vi "Periodic Tasks.vi"() -> ()   [LabVIEW 2011]
doc: "This VI runs in parallel to other tasks. It can contain as many user-defined periodic loops as you need. These can carry out PID or other sorts of timed response."
uses:
  <vilib>/Rock Robotics/SystemInterfaces/Utilities/FPGA_UtilitiesLED State.ctl
  <vilib>/Rock Robotics/SystemInterfaces/Utilities/FPGA_UtilitiesLED Source.ctl
  <vilib>/Rock Robotics/WPI/Relay/WPI_RelayValue.ctl
  Robot Global Data.vi
panel:
  out "Sent?":string="File Wrote"
  out "Voltage":dbl
  in  "Recording Array":dbl[][](array[numeric])
  in  "Turn on Record 2":bool
  out "Auton Recording 2":bool
  in  "Home Speed 2":dbl=1.0
  out "Ramp ACT Pot 2":dbl
  out "Auton Recording":bool
  in  "Turn on Record":bool
  in  "Auton Array":dbl[][](array[numeric])
  out "Right Rate":dbl
  out "Right Direction":bool
  out "Right Distance":dbl
  out "Shooter Encoder Distance":dbl
  out "Shooter Direction":bool
  out "Shooter Encoder Rate":dbl
  out "Left Rate":dbl
  out "Gyro Rate":dbl
  out "Gyro Angle":dbl
  out "Left Direction":bool
  out "Left Distance":dbl
  # "Auton Recording"
  # "Sensor Feedback"
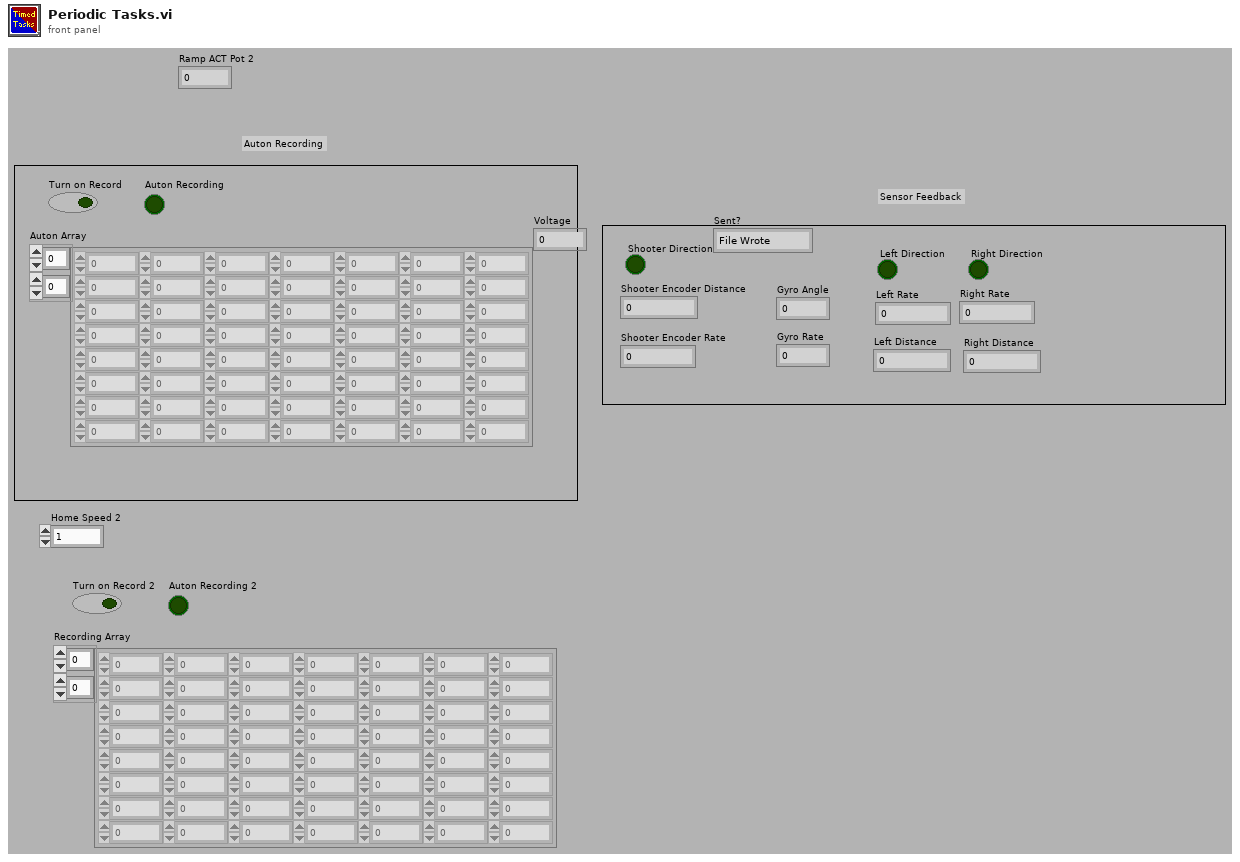
[diagram p1: front panel]
types:
  T1 = typedef "WPI_RelayValue.ctl" = enum16{"Off", "On", "Forward", "Reverse"}
  T2 = cluster{"Driver Station Digital Input (1-8)[0]":bool, "Driver Station Digital Input (1-8)[1]":bool, "Driver Station Digital Input (1-8)[2]":bool, "Driver Station Digital Input (1-8)[3]":bool, "Driver Station Digital Input (1-8)[4]":bool, "Driver Station Digital Input (1-8)[5]":bool, "Driver Station Digital Input (1-8)[6]":bool, "Driver Station Digital Input (1-8)[7]":bool, "Driver Station Digital Input (1-8)[8]":bool}
  T3 = typedef "WPI_AnalogChannelDevRef.ctl" = cluster{"DevStatus":errorcluster, "Analog Module":T4, "Analog Channel":T5}
  T4 = typedef "FPGA_TypedefAnalogModule.ctl" = enum16{"Analog Module 1", "Analog Module 2"}
  T5 = typedef "FPGA_AIChannel.ctl" = enum8{"AI 1", "AI 2", "AI 3", "AI 4", "AI 5", "AI 6", "AI 7", "AI 8", "Invalid"}
  T6 = typedef "WPI_EncoderDevRef.ctl" = cluster{"DevStatus":errorcluster, "EncoderIndex":T7, "CounterIndex":T8, "DistancePerCount":dbl, "Decoding Type":T9}
  T7 = typedef "FPGA_EncoderIdx.ctl" = enum8{"Enc 0", "Enc 1", "Enc 2", "Enc 3", "Invalid"}
  T8 = typedef "FPGA_CounterCtrSystemIndex.ctl" = enum8{"Ctr 0", "Ctr 1", "Ctr 2", "Ctr 3", "Ctr 4", "Ctr 5", "Ctr 6", "Ctr 7", "Invalid"}
  T9 = typedef "WPI_EncoderType.ctl" = enum16{"1x", "2x", "4x"}
  T10 = typedef "WPI_GyroDevRef.ctl" = cluster{"DevStatus":errorcluster, "Analog Module":T4, "Analog Channel":T5, "Offset":dbl, "Gain (VoltsPerDegree/Second)":dbl}
  T11 = typedef "WPI_RelayDevRef.ctl" = cluster{"DevStatus":errorcluster, "Relay Channel":T12, "Digital Module":T13, "Relay Direction":T14}
  T12 = typedef "FPGA_DIORelayChannel.ctl" = enum8{"Relay 1", "Relay 2", "Relay 3", "Relay 4", "Relay 5", "Relay 6", "Relay 7", "Relay 8", "Invalid"}
  T13 = typedef "FPGA_TypedefDigitalModule.ctl" = enum16{"Digital Module 1", "Digital Module 2"}
  T14 = typedef "WPI_RelayDirection.ctl" = enum16{"Both directions", "Forward only", "Reverse only"}
  T15 = typedef "FPGA_UtilitiesLED State.ctl" = enum16{"Off", "On", "Toggle"}
  T16 = typedef "FPGA_UtilitiesLED Source.ctl" = enum16{"User LED", "FPGA LED"}
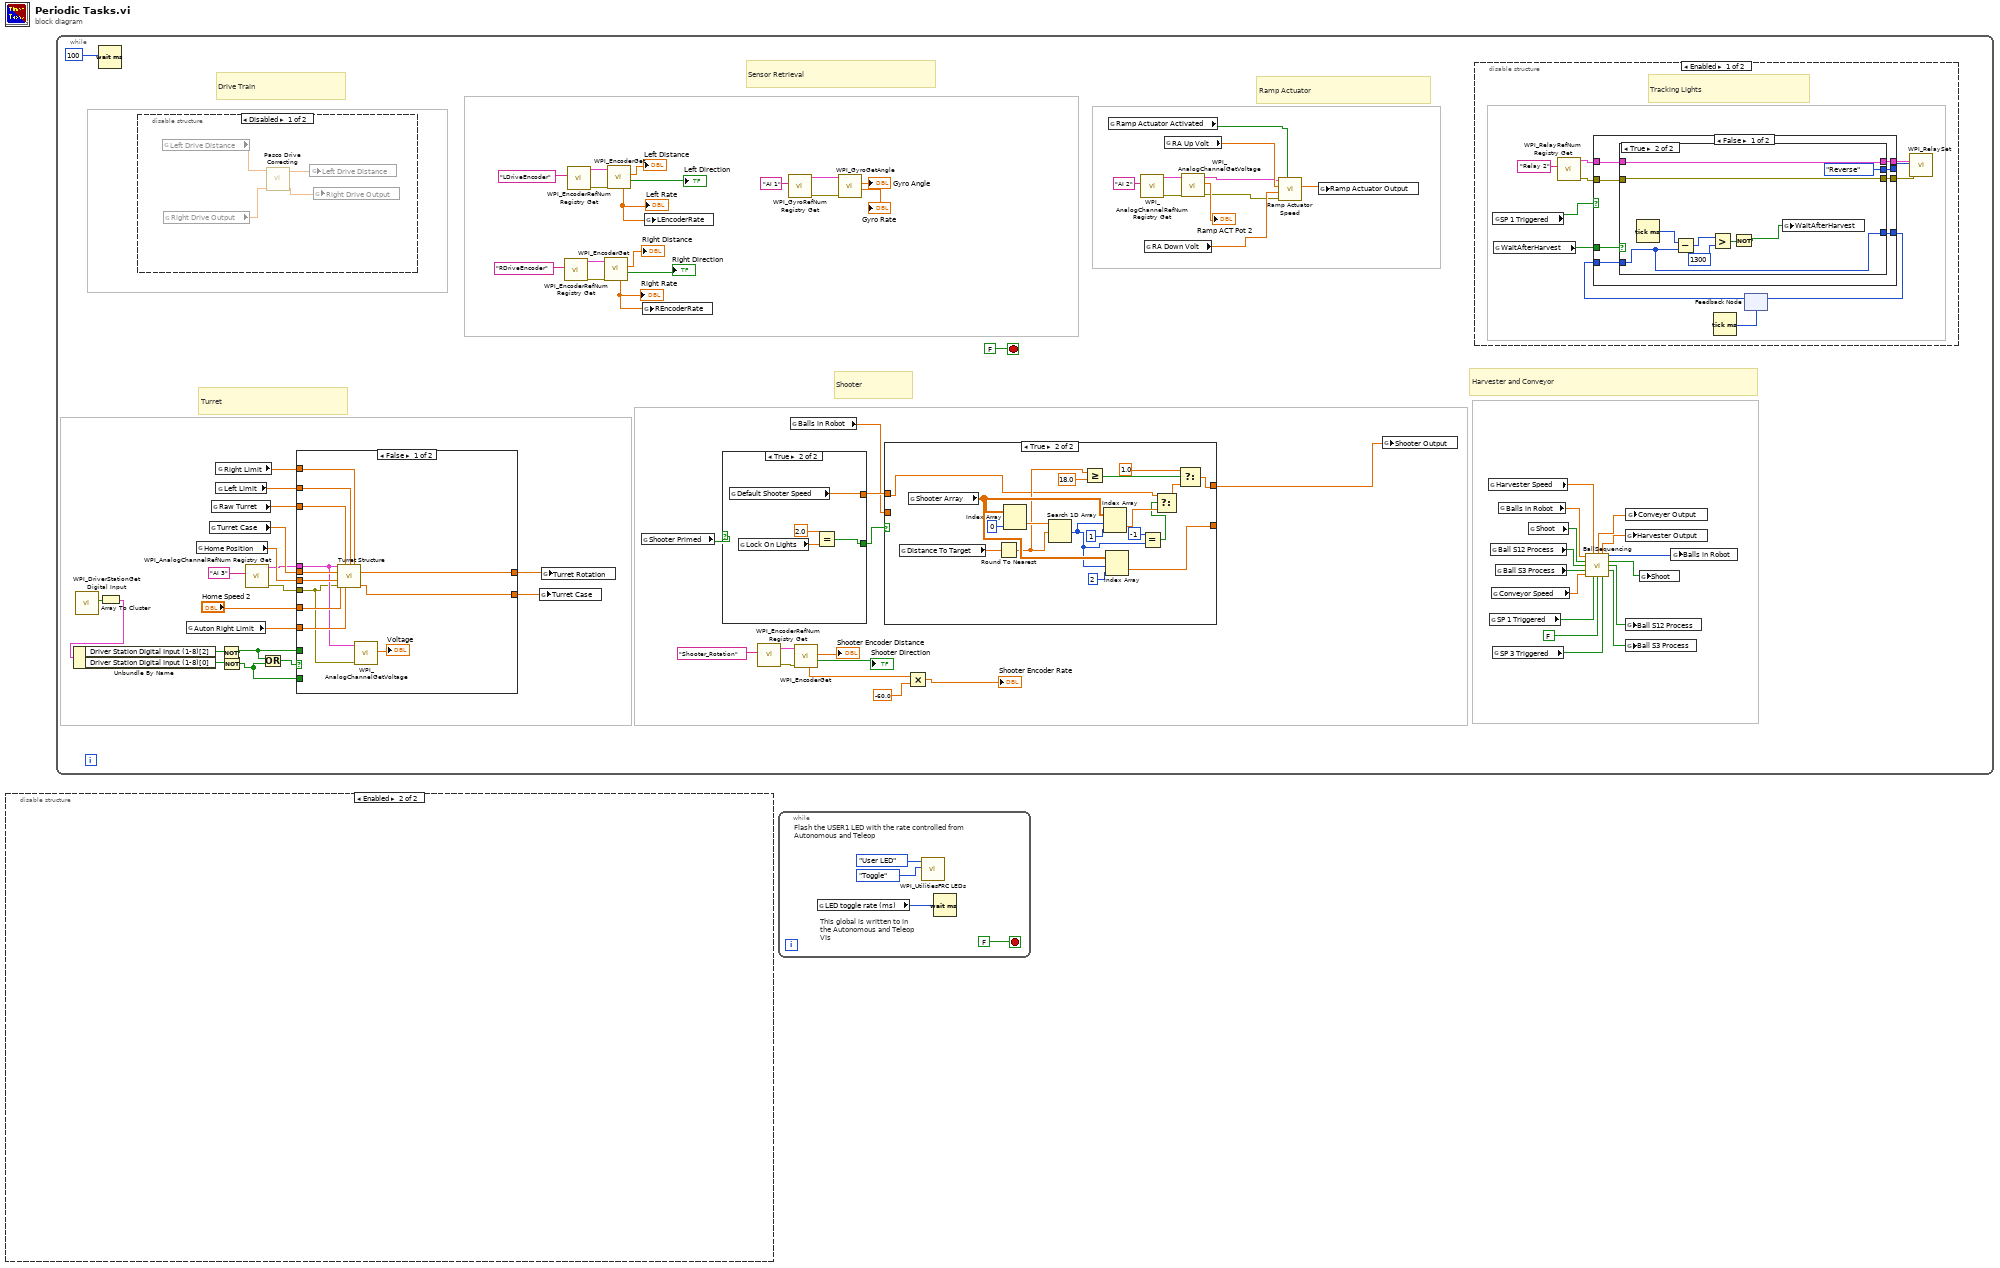
[diagram p0: block diagram]
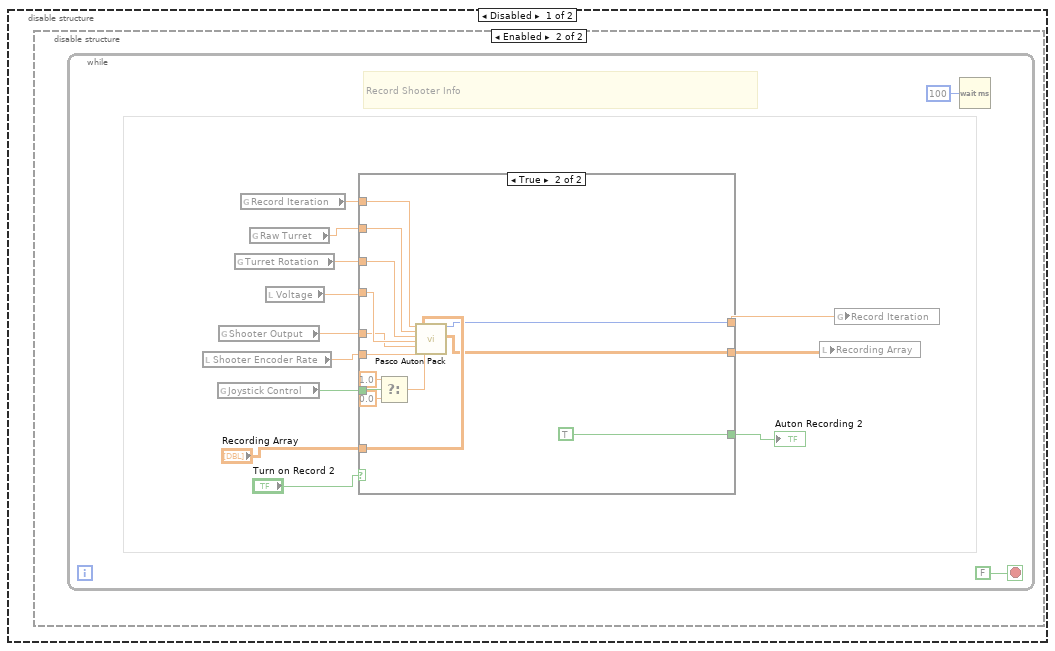
[diagram p2: hidden frame]
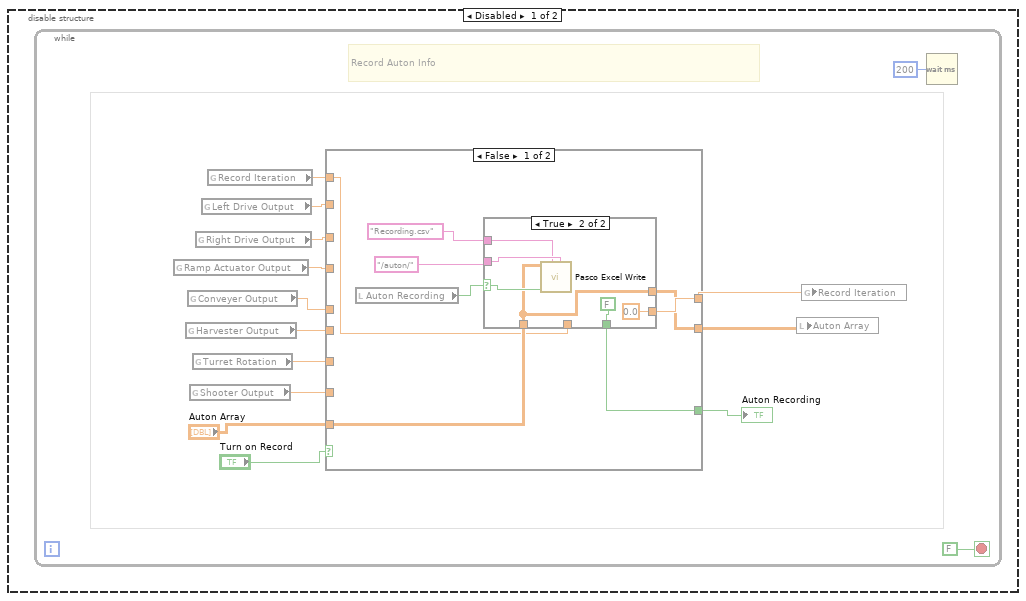
[diagram p3: hidden frame]
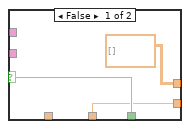
[diagram p4: hidden frame]
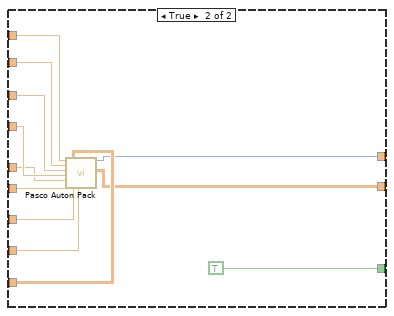
[diagram p5: hidden frame]
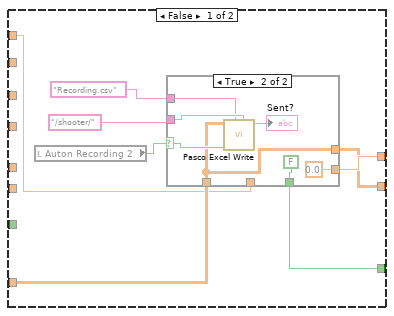
[diagram p6: hidden frame]
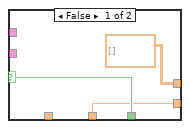
[diagram p7: hidden frame]
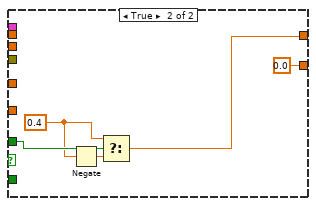
[diagram p8: hidden frame]
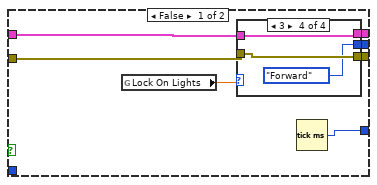
[diagram p9: hidden frame]
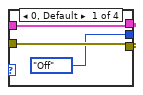
[diagram p10: hidden frame]
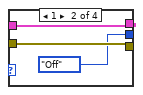
[diagram p11: hidden frame]
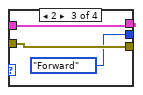
[diagram p12: hidden frame]
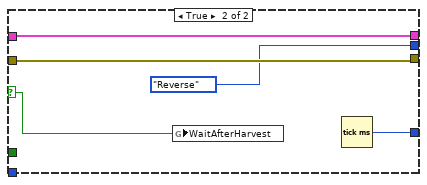
[diagram p13: hidden frame]
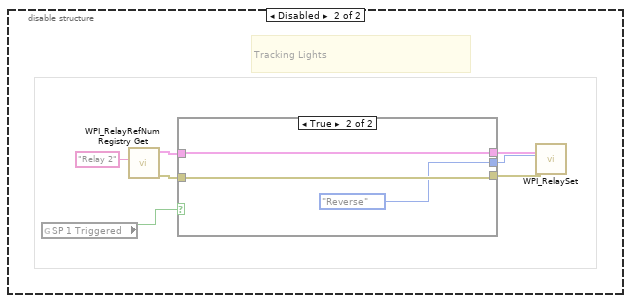
[diagram p14: hidden frame]
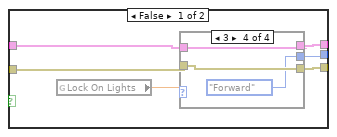
[diagram p15: hidden frame]
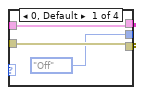
[diagram p16: hidden frame]
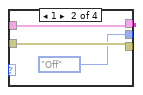
[diagram p17: hidden frame]
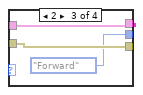
[diagram p18: hidden frame]
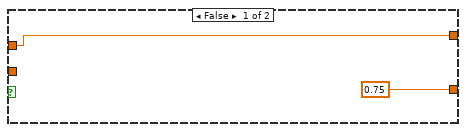
[diagram p19: hidden frame]
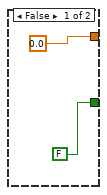
[diagram p20: hidden frame]
diagram:
  n1 = disable-structure shown="Enabled" {
    frame Disabled {
      n2 = disable-structure shown="Enabled" {
        frame Disabled {
          n3 = while {
            stop <- FALSE stop-if-true
            # "Record Auton Info"
            n4 = global read "Robot Global Data.vi" "Ramp Actuator Output"() -> (w5:dbl)
            n5 = global read "Robot Global Data.vi" "Harvester Output"() -> (w7:dbl)
            n6 = global read "Robot Global Data.vi" "Conveyer Output"() -> (w6:dbl)
            n7 = global read "Robot Global Data.vi" "Shooter Output"() -> (w9:dbl)
            n8 = global read "Robot Global Data.vi" "Turret Rotation"() -> (w8:dbl)
            n9 = global read "Robot Global Data.vi" "Right Drive Output"() -> (w4:dbl)
            n10 = global read "Robot Global Data.vi" "Left Drive Output"() -> (w3:dbl)
            n11 = global read "Robot Global Data.vi" "Record Iteration"() -> (w2:dbl)
            n12 = case shown="False" "Turn on Record" {
              tunnel: w2 -> [w19 w44]
              tunnel: w3 -> [_ w43]
              tunnel: w4 -> [_ w42]
              tunnel: w5 -> [_ w41]
              tunnel: w6 -> [_ w40]
              tunnel: w7 -> [_ w39]
              tunnel: w8 -> [_ w38]
              tunnel: w9 -> [_ w37]
              tunnel: "Auton Array" -> [w20 w36]
              tunnel: [w16 w35] -> w12
              tunnel: [w17 w34] -> w13
              tunnel: [w18 TRUE] -> w14
              frame False {
                n13 = local read "Auton Recording"() -> (w21:bool)
                n14 = case shown="True" w21 {
                  selector: w21 -> [w26 w31]
                  tunnel: [w26 FALSE] -> w18
                  tunnel: "/auton/" ("File Name") -> [_ w30]
                  tunnel: "Recording.csv" ("Folder Location") -> [_ w29]
                  tunnel: [w25 0.0 ("Record Iteration")] -> w17
                  tunnel: w19 -> [w25 _]
                  tunnel: w20 -> [_ w27]
                  tunnel: [dbl[][] [] ("Auton Array") w27] -> w16
                  frame False {
                  }
                  frame True {
                    n15 = call "Pasco Excel Write.vi"("Folder Location"=w30, "File Name"=w29, "WriteToExcel"=w31, "2D data"=w27) -> ()  [unwired: 7 in, 1 out]
                  }
                }
              }
              frame True {
                n16 = call "Pasco Auton Pack.vi"("Iterations"=w44, "Left Drive"=w43, "Right Drive"=w42, "RAMP ACT"=w41, "Conveyor"=w40, "Harvestor"=w39, "Auton Array"=w36, "Turret"=w38, "Shooter"=w37) -> ("Iteration Output"=w34:i32, "output array"=w35:dbl[][])  [unwired: 9 in]
              }
            }
            "Auton Recording" <- w14
            n17 = local write "Auton Array"(w12) -> ()
            n18 = global write "Robot Global Data.vi" "Record Iteration"(w13) -> ()
            n19 = Wait (ms)(milliseconds to wait=u32 200) -> ()  [unwired: 1 out]
          }
        }
        frame Enabled {
          n20 = while {
            stop <- FALSE stop-if-true
            # "Record Shooter Info"
            n21 = local read "Shooter Encoder Rate"() -> (w46:dbl)
            n22 = global read "Robot Global Data.vi" "Joystick Control"() -> (w45:bool)
            n23 = global read "Robot Global Data.vi" "Shooter Output"() -> (w47:dbl)
            n24 = global read "Robot Global Data.vi" "Turret Rotation"() -> (w49:dbl)
            n25 = global read "Robot Global Data.vi" "Record Iteration"() -> (w52:dbl)
            n26 = global read "Robot Global Data.vi" "Raw Turret"() -> (w50:dbl)
            n27 = local read "Voltage"() -> (w48:dbl)
            n28 = case shown="True" "Turn on Record 2" {
              tunnel: w52 -> [w62 w90]
              tunnel: w50 -> [_ w89]
              tunnel: w49 -> [_ w88]
              tunnel: w48 -> [_ w87]
              tunnel: w47 -> [_ w86]
              tunnel: w46 -> [_ w85]
              tunnel: "Recording Array" -> [w63 w84]
              tunnel: [w59 w83] -> w55
              tunnel: [w60 w82] -> w56
              tunnel: [w61 TRUE] -> w57
              tunnel: w45 -> [_ w80]
              frame False {
                n29 = local read "Auton Recording 2"() -> (w64:bool)
                n30 = case shown="True" w64 {
                  selector: w64 -> [w69 w75]
                  tunnel: [w69 FALSE] -> w61
                  tunnel: "/shooter/" ("File Name") -> [_ w74]
                  tunnel: "Recording.csv" ("Folder Location") -> [_ w73]
                  tunnel: [w68 0.0 ("Record Iteration")] -> w60
                  tunnel: w62 -> [w68 _]
                  tunnel: w63 -> [_ w71]
                  tunnel: [dbl[][] [] ("Auton Array") w71] -> w59
                  frame False {
                  }
                  frame True {
                    n31 = call "Pasco Excel Write.vi"("Folder Location"=w74, "File Name"=w73, "WriteToExcel"=w75, "2D data"=w71) -> ("Sent?"=→"Sent?":string)  [unwired: 7 in]
                  }
                }
              }
              frame True {
                n32 = Select(t=1.0, s=w80, f=0.0) -> (s? t:f=w77:dbl)
                n33 = call "Pasco Auton Pack.vi"("Iterations"=w90, "Left Drive"=w89, "Right Drive"=w88, "RAMP ACT"=w87, "Conveyor"=w86, "Harvestor"=w85, "Auton Array"=w84, "Turret"=w77) -> ("Iteration Output"=w82:i32, "output array"=w83:dbl[][])  [unwired: 10 in]
              }
            }
            "Auton Recording 2" <- w57
            n34 = local write "Recording Array"(w55) -> ()
            n35 = global write "Robot Global Data.vi" "Record Iteration"(w56) -> ()
            n36 = Wait (ms)(milliseconds to wait=u32 100) -> ()  [unwired: 1 out]
          }
        }
      }
    }
    frame Enabled {
    }
  }
  n37 = while {
    stop <- FALSE stop-if-true
    # "Harvester and Conveyor"
    # "Shooter"
    # "Sensor Retrieval"
    # "Turret"
    # "Drive Train"
    # "Ramp Actuator"
    n38 = call <vilib>:"WPI_DriverStationGet Digital Input.vi"() -> ("Driver Station Digital Input (1-8)"=w109:bool[])  [unwired: 11 in]
    n39 = Wait (ms)(milliseconds to wait=u32 100) -> ()  [unwired: 1 out]
    n40 = Array To Cluster(array=w109) -> (cluster=w108:T2)
    n41 = Unbundle By Name(w108) -> ("Driver Station Digital Input (1-8)[2]"=w94:bool, "Driver Station Digital Input (1-8)[0]"=w92:bool)
    n42 = disable-structure shown="Disabled" {
      frame Disabled {
        n43 = global read "Robot Global Data.vi" "Left Drive Distance"() -> (w293:dbl)
        n44 = global read "Robot Global Data.vi" "Right Drive Output"() -> (w292:dbl)
        n45 = call "Pasco Drive Correcting.vi"("RightDriveOutput"=w292, "LeftDriveOutput"=w293) -> ("RightDriveOutput"=w290:dbl, "LeftDriveOutput"=w291:dbl)  [unwired: 8 in]
        n46 = global write "Robot Global Data.vi" "Left Drive Distance"(w291) -> ()
        n47 = global write "Robot Global Data.vi" "Right Drive Output"(w290) -> ()
      }
      frame Enabled {
      }
    }
    n48 = global read "Robot Global Data.vi" "Auton Right Limit"() -> (w105:dbl)
    n49 = global read "Robot Global Data.vi" "Home Position"() -> (w100:dbl)
    n50 = global read "Robot Global Data.vi" "Turret Case"() -> (w99:dbl)
    n51 = global read "Robot Global Data.vi" "Raw Turret"() -> (w101:dbl)
    n52 = global read "Robot Global Data.vi" "Right Limit"() -> (w104:dbl)
    n53 = global read "Robot Global Data.vi" "Left Limit"() -> (w103:dbl)
    n54 = Not(x=w94) -> (.not. x?=w93:bool)
    n55 = Not(x=w92) -> (.not. x?=w91:bool)
    n56 = call <vilib>:"WPI_AnalogChannelRefNum Registry Get.vi"("refnum name"="AI 3") -> ("error out"=w98:errorcluster, "AIDeviceRef"=w97:T3)  [unwired: 9 in]
    n57 = Or(x=w93, y=w91) -> (x .or. y?=w95:bool)
    n58 = case shown="False" w95 {
      tunnel: w97 -> [w169 _]
      tunnel: w98 -> [w168 _]
      tunnel: w99 -> [w178 _]
      tunnel: w100 -> [w177 _]
      tunnel: w101 -> [w176 _]
      tunnel: "Home Speed 2" -> [w175 _]
      tunnel: w103 -> [w174 _]
      tunnel: w104 -> [w173 _]
      tunnel: w105 -> [w172 _]
      tunnel: [w171 w182] -> w106
      tunnel: [w170 0.0 ("Turret Case Output")] -> w107
      tunnel: w93 -> [_ w183]
      tunnel: w91 -> [_ _]
      frame False {
        n59 = call "Turret Structure.vi"("AIDeviceRef"=w169, "Raw Turret"=w176, "Left"=w174, "Right"=w173, "Turret Case"=w178, "Home Speed"=w175, "Home postion"=w177, "error in (no error)"=w168, "Auton Right"=w172) -> ("Turret Output"=w171:dbl, "Turret Case Output"=w170:dbl)  [unwired: 5 in]
        n60 = call <vilib>:"WPI_AnalogChannelGetVoltage.vi"("error in (no error)"=w168, "AIDeviceRef"=w169) -> ("Voltage"=→"Voltage":dbl)  [unwired: 7 in, 2 out]
      }
      frame True {
        w179 = 0.4 ("t")
        n61 = Negate(x=w179) -> (-x=w180:dbl)
        n62 = Select(t=w179, s=w183, f=w180) -> (s? t:f=w182:dbl)
      }
    }
    n63 = global write "Robot Global Data.vi" "Turret Case"(w107) -> ()
    n64 = global write "Robot Global Data.vi" "Turret Rotation"(w106) -> ()
    n65 = call <vilib>:"WPI_EncoderRefNum Registry Get.vi"("refnum name"="RDriveEncoder") -> ("error out"=w133:errorcluster, "EncoderDevRef"=w132:T6)  [unwired: 9 in]
    n66 = call <vilib>:"WPI_EncoderRefNum Registry Get.vi"("refnum name"="LDriveEncoder") -> ("error out"=w139:errorcluster, "EncoderDevRef"=w138:T6)  [unwired: 9 in]
    n67 = call <vilib>:"WPI_EncoderGet.vi"("error in (no error)"=w133, "EncoderDevRef"=w132) -> ("Direction"=→"Right Direction":bool, "Distance"=→"Right Distance":dbl, "Rate"=w129:dbl)  [unwired: 4 in, 3 out]
    "Right Rate" <- w129
    n68 = call <vilib>:"WPI_EncoderGet.vi"("error in (no error)"=w139, "EncoderDevRef"=w138) -> ("Direction"=→"Left Direction":bool, "Distance"=→"Left Distance":dbl, "Rate"=w135:dbl)  [unwired: 4 in, 3 out]
    "Left Rate" <- w135
    n69 = global read "Robot Global Data.vi" "Shooter Primed"() -> (w153:bool)
    n70 = global write "Robot Global Data.vi" "REncoderRate"(w129) -> ()
    n71 = global write "Robot Global Data.vi" "LEncoderRate"(w135) -> ()
    n72 = case shown="True" w153 {
      tunnel: [FALSE ("Shooter Primed") w287] -> w111
      tunnel: [0.0 w286] -> w151
      frame False {
      }
      frame True {
        n73 = global read "Robot Global Data.vi" "Default Shooter Speed"() -> (w286:dbl)
        n74 = global read "Robot Global Data.vi" "Lock On Lights"() -> (w289:dbl)
        n75 = Equal?(x=2.0, y=w289) -> (x = y?=w287:bool)
      }
    }
    n76 = call <vilib>:"WPI_EncoderRefNum Registry Get.vi"("refnum name"="Shooter_Rotation") -> ("error out"=w113:errorcluster, "EncoderDevRef"=w114:T6)  [unwired: 9 in]
    n77 = call <vilib>:"WPI_GyroRefNum Registry Get.vi"("refnum name"="AI 1") -> ("error out"=w147:errorcluster, "GyroDevRef"=w148:T10)  [unwired: 9 in]
    n78 = global read "Robot Global Data.vi" "Balls in Robot"() -> (w150:dbl)
    n79 = call <vilib>:"WPI_EncoderGet.vi"("error in (no error)"=w113, "EncoderDevRef"=w114) -> ("Direction"=→"Shooter Direction":bool, "Distance"=→"Shooter Encoder Distance":dbl, "Rate"=w110:dbl)  [unwired: 4 in, 3 out]
    n80 = call <vilib>:"WPI_GyroGetAngle.vi"("error in (no error)"=w147, "GyroDevRef"=w148) -> ("Angular Rate"=→"Gyro Rate":dbl, "Angle"=→"Gyro Angle":dbl)  [unwired: 6 in, 2 out]
    n81 = case shown="True" w111 {
      tunnel: [w265 w274] -> w152
      tunnel: w151 -> [w265 w266]
      tunnel: w150 -> [_ _]
      tunnel: [0.75 w283] -> _
      frame False {
      }
      frame True {
        n82 = global read "Robot Global Data.vi" "Distance To Target"() -> (w280:dbl)
        n83 = global read "Robot Global Data.vi" "Shooter Array"() -> (w277:dbl[][])
        n84 = Round To Nearest(number=w280) -> (nearest integer value=w275:dbl)
        n85 = Index Array(array=w277, index (col)=0 ("disabled index (col)")) -> (element=w279:dbl[])  [unwired: 1 in]
        n86 = Search 1D Array(1D array=w279, element=w275) -> (index of element=w269:i32)  [unwired: 1 in]
        n87 = Greater Or Equal?(x=w275, y=18.0) -> (x >= y?=w273:bool)
        n88 = Index Array(array=w277, index (row)=w269, index (col)=1 ("disabled index (col)")) -> (element=w270:dbl)
        n89 = Index Array(array=w277, index (row)=w269, index (col)=2 ("disabled index (col)")) -> (element=w283:dbl)
        n90 = Equal?(x=-1, y=w269) -> (x = y?=w267:bool)
        n91 = Select(t=w266, s=w267, f=w270) -> (s? t:f=w271:dbl)
        n92 = Select(t=1.0, s=w273, f=w271) -> (s? t:f=w274:dbl)
      }
    }
    n93 = Multiply(x=w110, y=-60.0) -> (x*y=→"Shooter Encoder Rate":dbl)
    n94 = global read "Robot Global Data.vi" "Ramp Actuator Activated"() -> (w124:bool)
    n95 = call <vilib>:"WPI_AnalogChannelRefNum Registry Get.vi"("refnum name"="AI 2") -> ("error out"=w122:errorcluster, "AIDeviceRef"=w123:T3)  [unwired: 9 in]
    n96 = global read "Robot Global Data.vi" "RA Down Volt"() -> (w127:dbl)
    n97 = global read "Robot Global Data.vi" "RA Up Volt"() -> (w126:dbl)
    n98 = call <vilib>:"WPI_AnalogChannelGetVoltage.vi"("error in (no error)"=w122, "AIDeviceRef"=w123) -> ("error out"=w119:errorcluster, "Voltage"=→"Ramp ACT Pot 2":dbl, "AIDeviceRef"=w120:T3)  [unwired: 7 in]
    n99 = call "Ramp Actuator Speed.vi"("Up to Down"=w124, "error in (no error)"=w119, "RA Down Volt"=w127, "RA Up Volt"=w126, "AIDeviceRef"=w120) -> ("Ramp Actuator Ouput"=w125:dbl)  [unwired: 6 in]
    n100 = global write "Robot Global Data.vi" "Ramp Actuator Output"(w125) -> ()
    n101 = global write "Robot Global Data.vi" "Shooter Output"(w152) -> ()
    n102 = disable-structure shown="Enabled" {
      frame Enabled {
        # "Tracking Lights"
        n103 = global read "Robot Global Data.vi" "SP 1 Triggered"() -> (w194:bool)
        n104 = global read "Robot Global Data.vi" "WaitAfterHarvest"() -> (w187:bool)
        n105 = call <vilib>:"WPI_RelayRefNum Registry Get.vi"("refnum name"="Relay 2") -> ("error out"=w192:errorcluster, "RelayDevRef"=w190:T11)  [unwired: 9 in]
        n106 = Tick Count (ms)() -> (millisecond timer value=w184:u32)
        n107 = feedback #1(w184) -> (w185:u32)
        n108 = case shown="False" w194 {
          selector: w194 -> [_ w232]
          tunnel: [w202 w235] -> w189
          tunnel: w190 -> [w201 w235]
          tunnel: [w200 w234] -> w191
          tunnel: w192 -> [w199 w234]
          tunnel: [w198 WPI_RelayValue."Reverse" ("RelayValue")] -> w193
          tunnel: [w195 w231] -> w186
          tunnel: w187 -> [w197 _]
          tunnel: w185 -> [w196 _]
          frame False {
            n109 = case shown="True" w197 {
              tunnel: [w209 w230] -> w202
              tunnel: w201 -> [w208 w230]
              tunnel: [w207 w229] -> w200
              tunnel: w199 -> [w206 w229]
              tunnel: [w205 WPI_RelayValue."Reverse" ("RelayValue")] -> w198
              tunnel: w196 -> [_ w222]
              tunnel: [w203 w222] -> w195
              frame False {
                n110 = global read "Robot Global Data.vi" "Lock On Lights"() -> (w204:dbl)
                n111 = case shown="3" w204 {
                  tunnel: [w212 w215 w218 w221] -> w209
                  tunnel: w208 -> [w212 w215 w218 w221]
                  tunnel: [w211 w214 w217 w220] -> w207
                  tunnel: w206 -> [w211 w214 w217 w220]
                  tunnel: [WPI_RelayValue."Off" ("RelayValue") WPI_RelayValue."Off" ("RelayValue") WPI_RelayValue."Forward" ("RelayValue") WPI_RelayValue."Forward" ("RelayValue")] -> w205
                  frame 0, Default {
                  }
                  frame 1 {
                  }
                  frame 2 {
                  }
                  frame 3 {
                  }
                }
                n112 = Tick Count (ms)() -> (millisecond timer value=w203:u32)
              }
              frame True {
                n113 = Tick Count (ms)() -> (millisecond timer value=w227:u32)
                n114 = Subtract(x=w227, y=w222) -> (x-y=w226:u32)
                n115 = Greater?(x=w226, y=u32 1300) -> (0:w224:bool)
                n116 = Not(x=w224) -> (.not. x?=w223:bool)
                n117 = global write "Robot Global Data.vi" "WaitAfterHarvest"(w223) -> ()
              }
            }
          }
          frame True {
            n118 = global write "Robot Global Data.vi" "WaitAfterHarvest"(w232) -> ()
            n119 = Tick Count (ms)() -> (millisecond timer value=w231:u32)
          }
        }
        n120 = feedback-in #1(w186) -> ()
        n121 = call <vilib>:"WPI_RelaySet.vi"("error in (no error)"=w191, "RelayValue"=w193, "RelayDevRef"=w189) -> ()  [unwired: 7 in, 2 out]
      }
      frame Disabled {
        # "Tracking Lights"
        n122 = global read "Robot Global Data.vi" "SP 1 Triggered"() -> (w242:bool)
        n123 = call <vilib>:"WPI_RelayRefNum Registry Get.vi"("refnum name"="Relay 2") -> ("error out"=w240:errorcluster, "RelayDevRef"=w238:T11)  [unwired: 9 in]
        n124 = case shown="True" w242 {
          tunnel: [w248 w263] -> w237
          tunnel: w238 -> [w247 w263]
          tunnel: [w246 w262] -> w239
          tunnel: w240 -> [w245 w262]
          tunnel: [w244 WPI_RelayValue."Reverse" ("RelayValue")] -> w241
          frame False {
            n125 = global read "Robot Global Data.vi" "Lock On Lights"() -> (w243:dbl)
            n126 = case shown="3" w243 {
              tunnel: [w251 w254 w257 w260] -> w248
              tunnel: w247 -> [w251 w254 w257 w260]
              tunnel: [w250 w253 w256 w259] -> w246
              tunnel: w245 -> [w250 w253 w256 w259]
              tunnel: [WPI_RelayValue."Off" ("RelayValue") WPI_RelayValue."Off" ("RelayValue") WPI_RelayValue."Forward" ("RelayValue") WPI_RelayValue."Forward" ("RelayValue")] -> w244
              frame 0, Default {
              }
              frame 1 {
              }
              frame 2 {
              }
              frame 3 {
              }
            }
          }
          frame True {
          }
        }
        n127 = call <vilib>:"WPI_RelaySet.vi"("error in (no error)"=w239, "RelayValue"=w241, "RelayDevRef"=w237) -> ()  [unwired: 7 in, 2 out]
      }
    }
    n128 = global read "Robot Global Data.vi" "Harvester Speed"() -> (w149:dbl)
    n129 = global read "Robot Global Data.vi" "SP 1 Triggered"() -> (w156:bool)
    n130 = global read "Robot Global Data.vi" "Ball S12 Process"() -> (w158:bool)
    n131 = global read "Robot Global Data.vi" "Conveyor Speed"() -> (w141:dbl)
    n132 = global read "Robot Global Data.vi" "SP 3 Triggered"() -> (w155:bool)
    n133 = global read "Robot Global Data.vi" "Ball S3 Process"() -> (w157:bool)
    n134 = global read "Robot Global Data.vi" "Balls in Robot"() -> (w160:dbl)
    n135 = global read "Robot Global Data.vi" "Shoot"() -> (w159:bool)
    n136 = call "BallSequencing.vi"("Balls In Robot"=w160, "Speed of Harvester"=w149, "Shoot"=w159, "Ball S12 Process"=w158, "Ball S3 Process"=w157, "Speed of Conveyor"=w141, "SP 1 Triggered"=w156, "SP 2 Triggered"=FALSE, "SP 3 Triggered"=w155) -> ("Conveyer Output"=w161:dbl, "Harvester Output"=w162:dbl, "Balls In Robot Output"=w143:i32, "Shoot Output"=w142:bool, "Ball S12 Process Output"=w164:bool, "Ball S3 Process Output"=w163:bool)  [unwired: 1 in]
    n137 = global write "Robot Global Data.vi" "Harvester Output"(w162) -> ()
    n138 = global write "Robot Global Data.vi" "Ball S12 Process"(w164) -> ()
    n139 = global write "Robot Global Data.vi" "Ball S3 Process"(w163) -> ()
    n140 = global write "Robot Global Data.vi" "Conveyer Output"(w161) -> ()
    n141 = global write "Robot Global Data.vi" "Shoot"(w142) -> ()
    n142 = global write "Robot Global Data.vi" "Balls in Robot"(w143) -> ()
  }
  n143 = while {
    stop <- FALSE stop-if-true
    # "This global is written to in the Autonomous and Teleop VIs"
    # "Flash the USER1 LED with the rate controlled from Autonomous and Teleop"
    n144 = global read "Robot Global Data.vi" "LED toggle rate (ms)"() -> (w294:u32)
    n145 = call <vilib>:"WPI_UtilitiesFRC LEDs.vi"("State"=FPGA_UtilitiesLED_State."Toggle", "LED Type"=FPGA_UtilitiesLED_Source."User LED") -> ()  [unwired: 1 in, 9 out]
    n146 = Wait (ms)(milliseconds to wait=w294) -> ()  [unwired: 1 out]
  }
